vi "1D DST.vi"(10 "DST size":i32=-1, 11 "X":dbl[](array[numeric])) -> (0 "error":i32, 3 "DST {X}":dbl[](array[numeric]))   [LabVIEW 2020, in "NI_AALPro.lvlib"]
doc: "Computes the Discrete Sine Transform (DST) of the input sequence <B>X</B>. Wire data to the <B>X</B> input to determine the polymorphic instance to use or manually select the instance."
uses:
  NI_AALPro.lvlib
  <resource>/lvanlys.dll
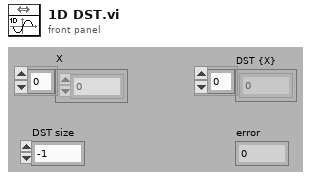
[diagram p1: front panel]
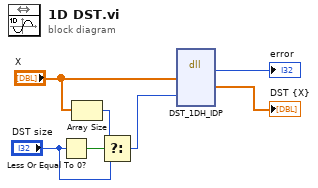
[diagram p0: block diagram]
diagram:
  n1 = Less Or Equal To 0?(x="DST size") -> (x <= 0?=w7:bool)
  n2 = Array Size(array="X") -> (size(s)=w4:i32)
  n3 = Select(t=w4, s=w7, f="DST size") -> (s? t:f=w3:i32)
  n4 = dll-call lib="C:/Program Files (x86)/National Instruments/LabVIEW 2020/resource/lvanlys.*" fn="DST_1DH_IDP"("xH"="X", "DCTSize"=w3) -> ("return type"=→"error":i32, "yH"=→"DST {X}":dbl[])  [unwired: 8 in, 2 out]
